vi "Generalized Eigenvalues and Vectors.vi"   [LabVIEW 2010, in "NI_AALPro.lvlib"]
doc: "Computes the generalized right eigenvalues and eigenvectors of the matrix pair <B>A</B> and <B>B</B>. The data types you wire to the <B>A</B> and <B>B</B> inputs determine the polymorphic instance to use."
uses:
  NI_AALPro.lvlib
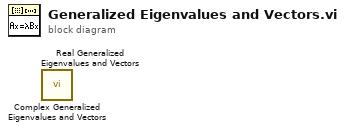
[diagram p0: block diagram]
diagram:
  n1 = call "Complex Generalized Eigenvalues and Vectors.vi"() -> ()  [unwired: 6 in, 3 out]
  n2 = call "Real Generalized Eigenvalues and Vectors.vi"() -> ()  [unwired: 6 in, 3 out]
